vi "ATF-Pump-GET FAIL SEQ FGV.vi"(8 "error in":errorcluster, 9 "Failure \ncase Seq":string[](array[string]), 11 "Enum":enum16{"Read", "Write "}(ring)) -> (0 "error out":errorcluster, 1 "Failure \ncase Seq":string[](array[string]))   [LabVIEW 2022 SP3]
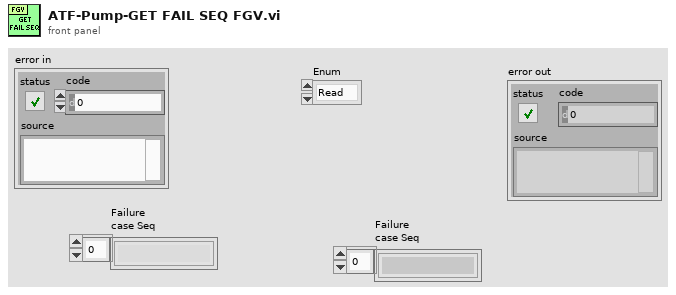
[diagram p1: front panel]
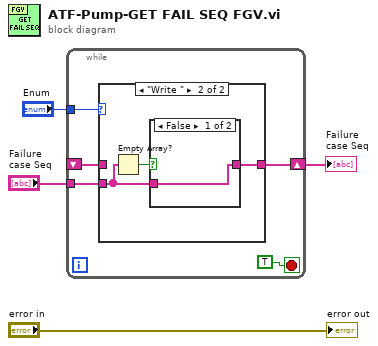
[diagram p0: block diagram]
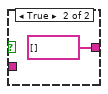
[diagram p3: hidden frame]
diagram:
  n1 = while {
    tunnel: "Enum" -> [w9]
    tunnel: "Failure \ncase Seq" -> [w7]
    shift-right: [w6] -> w1
    shift-left: _ -> [w5]
    stop <- TRUE stop-if-true
    n2 = case shown="\"Write \"" w9 {
      tunnel: w7 -> [_ w11]
      tunnel: [w10 w12] -> w6
      tunnel: w5 -> [w10 _]
      frame "Read", Default {
      }
      frame "Write " {
        n3 = Empty Array?(array=w11) -> (empty?=w13:bool)
        n4 = case shown="False" w13 {
          tunnel: [w14 string[] [] ("Failure \ncase Seq")] -> w12
          tunnel: w11 -> [w14 _]
          frame False {
          }
          frame True {
          }
        }
      }
    }
  }
  "Failure \ncase Seq" <- w1
  "error out" <- "error in"
